vi "ConsumeBefore.vi"(2 "error in":errorcluster {"code" format="%.0x"}, 3 "ASCII":bool, 4 "Before":string, 5 "Response String In":string) -> (0 "error out":errorcluster {"code" format="%.0x"}, 1 "Response String Out":string)   [LabVIEW 2010]
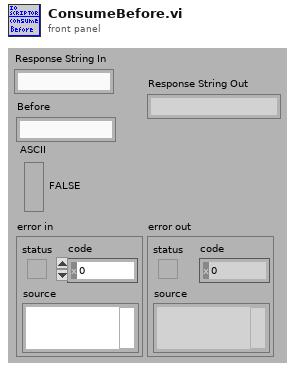
[diagram p1: front panel]
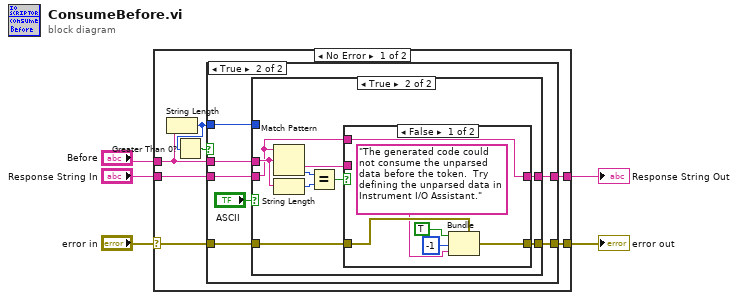
[diagram p0: block diagram]
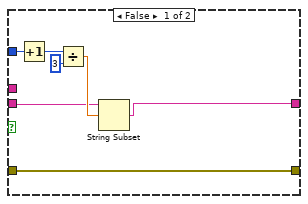
[diagram p3: hidden frame]
diagram:
  n1 = case shown="No Error" "error in" {
    selector: "error in" -> [w7 w47]
    tunnel: [w12 w46] -> w5
    tunnel: "Before" -> [w11 _]
    tunnel: "Response String In" -> [w10 w46]
    tunnel: [w6 w47] -> w1
    frame No Error {
      n2 = String Length(string=w11) -> (length=w9:i32)
      n3 = Greater Than 0?(x=w9) -> (x > 0?=w8:bool)
      n4 = case shown="True" w8 {
        tunnel: [w14 w21] -> w12
        tunnel: w9 -> [_ w20]
        tunnel: w11 -> [_ w19]
        tunnel: w10 -> [w14 w18]
        tunnel: w7 -> [w13 w16]
        tunnel: [w13 w15] -> w6
        frame False {
        }
        frame True {
          n5 = case shown="True" "ASCII" {
            tunnel: w18 -> [w24 w31]
            tunnel: [w26 w32] -> w21
            tunnel: w20 -> [w27 _]
            tunnel: w19 -> [_ w37]
            tunnel: w16 -> [w22 w30]
            tunnel: [w22 w29] -> w15
            frame False {
              n6 = Increment(x=w27) -> (x+1=w23:i32)
              n7 = Divide(x=w23, y=3) -> (x/y=w25:dbl)
              n8 = String Subset(string=w24, offset (0)=w25) -> (substring=w26:string)  [unwired: 1 in]
            }
            frame True {
              n9 = Match Pattern(string=w31, regular expression=w37) -> (after substring=w33:string, offset past match=w35:i32)  [unwired: 1 in, 2 out]
              n10 = String Length(string=w37) -> (length=w36:i32)
              n11 = Equal?(x=w35, y=w36) -> (x = y?=w34:bool)
              n12 = case shown="False" w34 {
                tunnel: w33 -> [_ w45]
                tunnel: [w43 w45] -> w32
                tunnel: w31 -> [w43 _]
                tunnel: w30 -> [w41 w44]
                tunnel: [w42 w44] -> w29
                frame False {
                  n13 = Bundle(cluster=w41, "status"=TRUE, "code"=-1, "source"="The generated code could not consume the unparsed data before the token.  Try defining the unparsed data in Instrument I/O Assistant.") -> (w42:errorcluster)
                }
                frame True {
                }
              }
            }
          }
        }
      }
    }
    frame Error {
    }
  }
  "Response String Out" <- w5
  "error out" <- w1
